vi "Display Queue Reference Handler.vi"(8 "Error In":errorcluster, 10 "Reference Action":T1, 11 "Queue Ref In":refnum<queue>) -> (0 "Error Out":errorcluster, 3 "Queue Ref Out":refnum<queue>)   [LabVIEW 2017]
uses:
  Reference Action.ctl
  Message Cluster.ctl
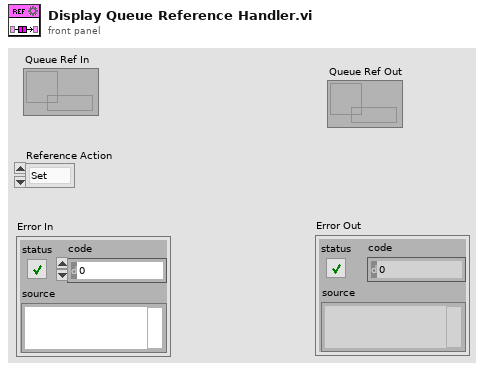
[diagram p1: front panel]
types:
  T1 = typedef "Reference Action.ctl" = enum16{"Set", "Get"}
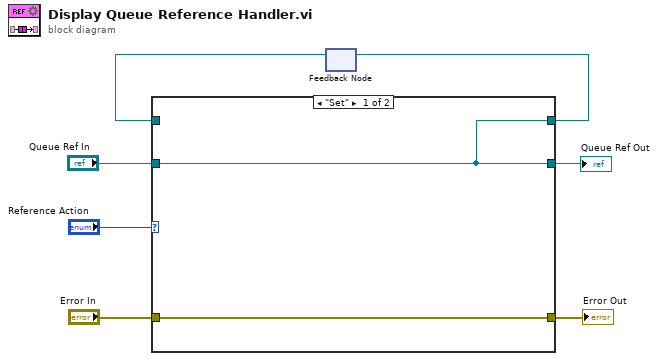
[diagram p0: block diagram]
diagram:
  n1 = feedback #1() -> (w5:refnum<queue>)  [unwired: 1 in]
  n2 = case shown="\"Set\"" "Reference Action" {
    tunnel: "Queue Ref In" -> [w9 _]
    tunnel: [w9 w11] -> w1
    tunnel: [w9 w11] -> w6
    tunnel: w5 -> [_ w11]
    tunnel: [w8 w10] -> w3
    tunnel: "Error In" -> [w8 w10]
    frame "Set" {
    }
    frame "Get", Default {
    }
  }
  "Error Out" <- w3
  "Queue Ref Out" <- w1
  n3 = feedback-in #1(w6) -> ()
